vi "Maxi Gauge-Clear Buffer.vi"(7 "W/R":bool, 8 "Fehler (Eingang)":errorcluster, 10 "Node address":u8, 11 "VISA-Ressource in":refnum<visa-resource-name>) -> (0 "Fehler (Ausgang)":errorcluster, 3 "VISA-Ressource out":refnum<visa-resource-name>)   [LabVIEW 2013, in "Maxi Gauge.lvlib"]
uses:
  <instrlib>/Maxi Gauge/Maxi Gauge.lvlib
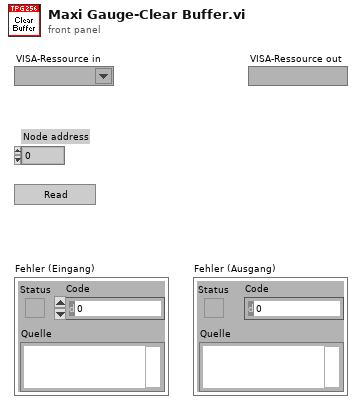
[diagram p1: front panel]
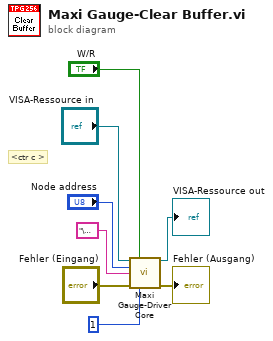
[diagram p0: block diagram]
diagram:
  # "<ctr c >"
  n1 = call <instrlib>:"Maxi Gauge-Driver Core.vi"("VISA-Ressource in"="VISA-Ressource in", "Write/Read"="W/R", "Node address"="Node address", "Command"="\u0003", "Fehler (Eingang)"="Fehler (Eingang)", "Timeout [ms]"=u32 1) -> ("VISA-Ressource out"=→"VISA-Ressource out":refnum<visa-resource-name>, "Fehler (Ausgang)"=→"Fehler (Ausgang)":errorcluster)  [unwired: 7 in, 1 out]
